vi "Main_v5.vi"() -> ()   [LabVIEW 2018]
uses:
  Clusters/FileDataChannel.ctl
  <vilib>/Platform/TimedLoop/XDataNode/timing_clust.ctl
  <vilib>/Platform/TimedLoop/XDataNode/nitl_modes.ctl
  <vilib>/Platform/TimedLoop/XDataNode/wakeup.ctl
  <vilib>/Analysis/Matrix/Datatypes/RealMatrix.ctl
  Clusters/ArrayPairs.ctl
  Clusters/SwapArrayCluster.ctl
  Clusters/RoscoParams.ctl
  Clusters/SimulationConstants.ctl
  Clusters/SwapIndexes.ctl
  <vilib>/Utility/file.llb/Read Delimited Spreadsheet (DBL).vi
  <vilib>/platform/TimedLoop/XDataNode/XDataNode.xnode
  <vilib>/Platform/TimedLoop/XDataNode/XDNodeRunTimeDep.lvlib
  <vilib>/Analysis/Matrix/NI_Matrix.lvlib
  <vilib>/ptbypt/NI_PtbyPt.lvlib
panel:
  out "error":i32
  in  "Config File Location":path=path "/home/lvuser/testcopy"
  out "Iteration Duration":i64
  out "Generator Speed (rad/s)":sgl(slide)=7.06858e-05 scale=-4.0..4.0
  in  "?":T1(tab)
  out "Generator Speed":sgl(graph)
  out "Torque Setpoint (Nm)":sgl(graph)
  out "Pitch Setpoint":sgl(graph)
  out "Aero Torque":dbl(graph)
  in  "GenSpeed Mean":sgl=10.0
  in  "GenSpeeed Amplitude":sgl=1.0
  out "windspeed":sgl(graph)
  out "Cp 2":dbl
  in  "GenSpeed Mean 2":sgl=3.0
  in  "GenSpeeed Amplitude 2":sgl=7.0
  out "Aero Torque  2":sgl(graph)
  in  "To VS_ControlMode":T2(ring)
  in  "Edit DISCON":bool
  out "DISCON.IN Contents":string
  in  "From VS_ControlMode":T2(ring)
  out "avrSWAP":sgl[](array[numeric])
  out "?":dbl
  out "Disp":dbl
  out "OUT_AEROTQ":sgl
  out "Cp array":dbl[][](array[numeric])
  out "Cp":dbl
  out "OUT_ROTSP":sgl
  out "OUT_DEBUG":sgl
  out "y(t)":dbl[](array[numeric]) format="%#_13g"
  out "thetadotdot/acc":dbl
  out "thetadot/vel":dbl
  out "Rotor Speed (rad/s)":sgl(slide)=7.06858e-05 scale=-4.0..4.0
  out "Torque Setpoint (kNm)":sgl(knob) scale=0.0..21586451.0
  out "Pitch Setpoint":sgl(knob) scale=0.0..1.5
  out "Power (kW)":sgl(slide) scale=0.0..20000000.0 scale format="%.2f"
  in  "Init WindSpeed(m/s)":sgl=7.0
  in  "File path":path=path "/home/lvuser/rosco-tests"
  out "SimLoop Late?":bool
  out "FIFO Loop Late?":bool
  in  "Base filename":string="rosco-tests"
  out "Writing to cRIO?":bool
  in  "WriteData":bool
  in  "?":T3
  out "#RT FIFO":u32
  out "Call to Rosco Failed?":bool
  out "Rosco Return Message":string
  in  "?":bool
  out "time(s)":dbl
  out "RT Loop Late?":bool
  # "FOCAL Realtime Control (IEA 15MW)"
  # "SENSOR INPUTS"
  # "FILEWRITING SETTINGS"
  # "ERRORS"
  # "TURBINE SPECIFICATIONS"
  # "ROSCO OUTPUTS"
  # "RATED POWER: 15000000 W"
  # "RATED TORQUE: 19624046.66 Nm"
  # "RATED GEN SPEED: 0.79168 rad/s"
  # "ROSCO INPUTS"
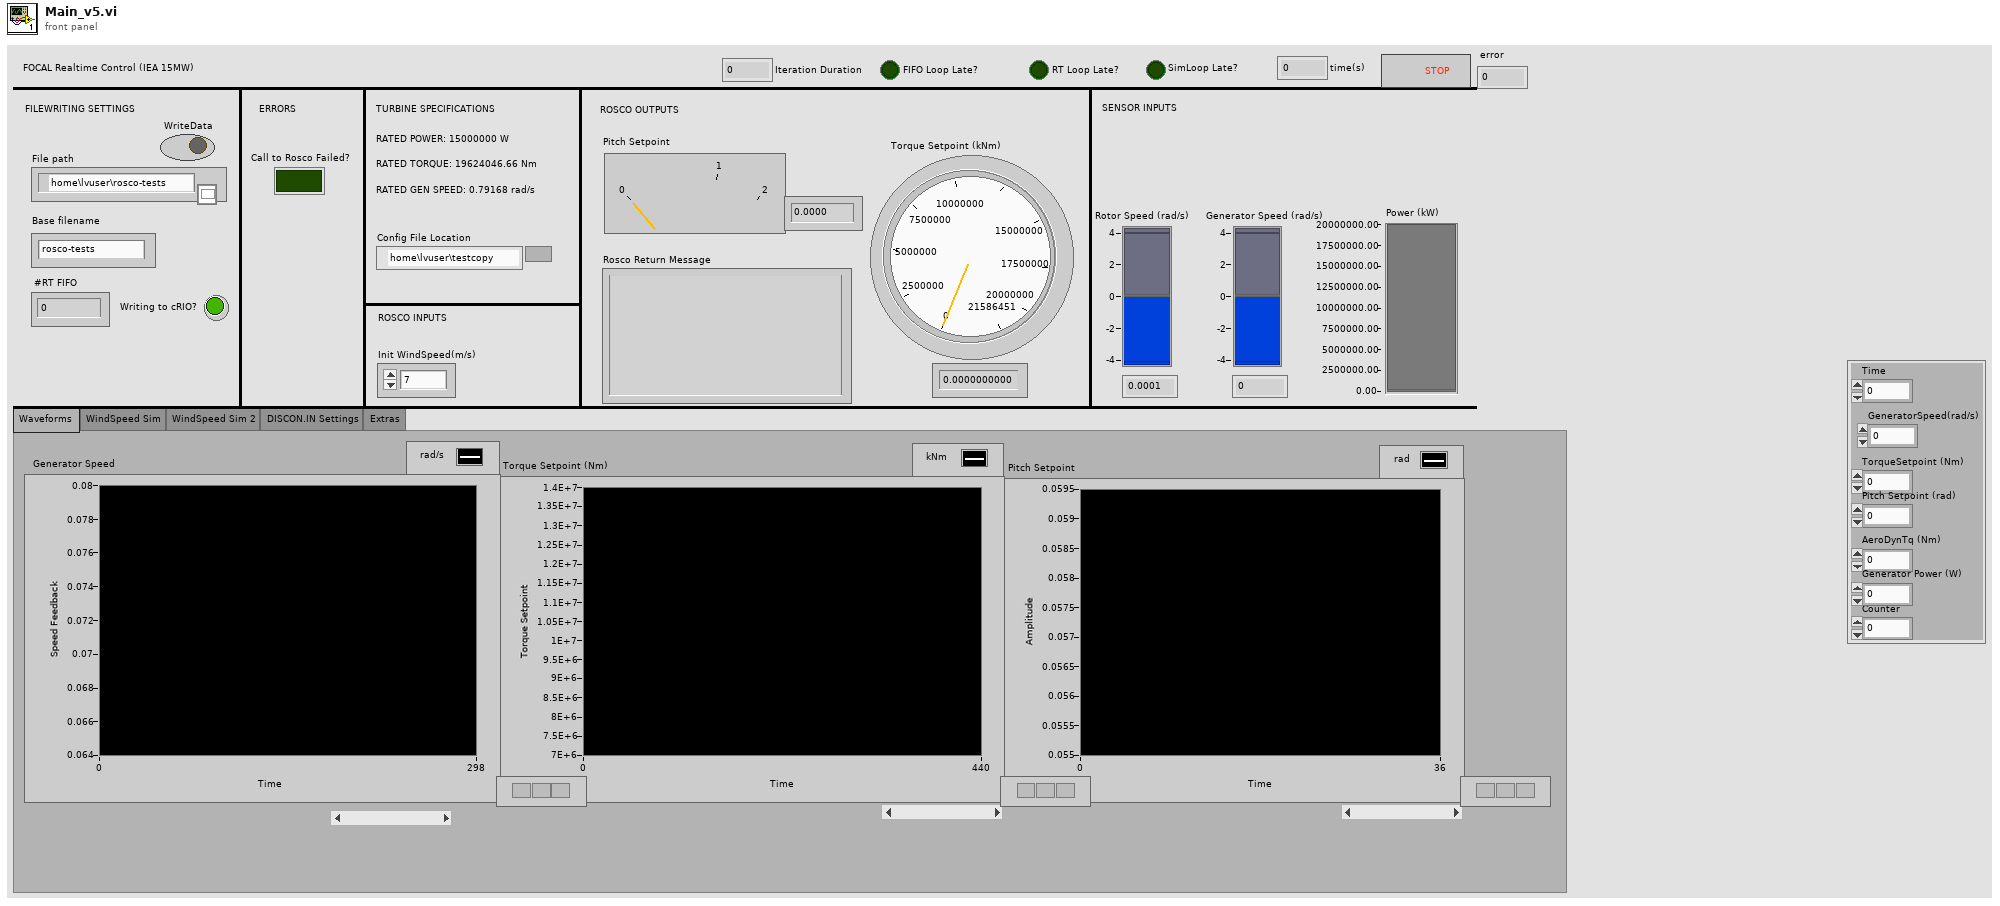
[diagram p1: front panel]
types:
  T1 = enum32{"Waveforms", "WindSpeed Sim", "WindSpeed Sim 2", "DISCON.IN Settings", "Extras"}
  T2 = enum16{"Constant Torque", "Constant Power", "PI Control"}
  T3 = typedef "FileDataChannel.ctl" = cluster{"GeneratorSpeed(rad/s)":sgl, "Counter":sgl, "Time":sgl, "TorqueSetpoint (Nm)":sgl, "Pitch Setpoint (rad)":sgl, "AeroDynTq (Nm) ":sgl, "Generator Power (W) ":sgl}
  T4 = typedef "NI_Matrix.lvlib/RealMatrix.ctl" = dbl[][]
  T5 = typedef "ArrayPairs.ctl" = cluster{"iStatus":T6, "TIME":T6, "DT":T6, "BL_PITCH":T6, "VS_MECHGENPWR":T6, "VS_GENPWR":T6, "GEN_SPEED":T6, "ROTOR_SPEED":T6, "GENTQMEAS":T6, "Y_M":T6, "HORWINDV":T6, "ROOTMOOP1":T6, "ROOTMOOP2":T6, "BL_PITCH2":T6, "BL_PITCH3":T6, "ROOTMOOP3":T6, "AVCMSG_SIZE":T6, "INFILE_SIZE ":T6, "OUTFILE_SIZE ":T6, "FA_ACC":T6, "NUM_BLADES":T6, "OUT_BL_PITCH":T6, "OUT_TORQUE":T6, "OUT_AEROTQ":T6, "Out.RotSpeed ":T6, "Out.DEBUG":T6}
  T6 = typedef "SwapArrayCluster.ctl" = cluster{"Index":i32, "Value":sgl}
  T7 = typedef "RoscoParams.ctl" = cluster{"avrSWAP":sgl[], "aviFAIL":i32, "avcMSG":string, "ReturnValue":i32}
  T8 = typedef "SwapIndexes.ctl" = cluster{"iSTATUS":i32, "TIME":i32, "DT":i32, "BL_PITCH_1":i32, "VS_MECHGENPWR":i32, "GEN_SPEED":i32, "ROT_SPEED":i32, "GENTQMEAS":i32, "Y_M":i32, "HORWINDV":i32, "ROOTMOOP1":i32, "ROOTMOOP2":i32, "BL_PITCH_2":i32, "BL_PITCH_3":i32, "ROOTMOOP3":i32, "INFILE_SIZE":i32, "FA_ACC":i32, "NUM_BLADES":i32, " OUT BL_PITCH":i32, "OUT_ TORQUE":i32, "OUTFILE_SIZE ":i32, "AVCMSG_SIZE":i32, "AERODYN TQ":i32, "VS_GENPWR":i32}
  T9 = typedef "XDNodeRunTimeDep.lvlib/timing_clust.ctl" = cluster{"Expected End [f-1]":u64, "Actual End [f-1]":u64, "Finished Late? [f-1]":bool, "Expected End [i-1]":u64, "Actual End [i-1]":u64, "Finished Late? [i-1]":bool, "Expected Start [i]":u64, "Actual Start [i]":u64, "Expected Start [f]":u64, "Actual Start [f]":u64, "Source Name":string, "Structure Name":string, "Period":i64, "Deadline":i64, "Offset":i64, "Start":i64, "Priority":i32, "Timeout":i32, "Mode":T10, "Wakeup Reason":T11, "Error":errorcluster, "Source Type":string, "Secondary Source Type":string, "Global End Time":u64, "Global Start Time":u64, "Frame Duration":u64, "Iteration Duration":u64, "Assigned CPU":i32, "I/O Scan Engine Mode":u32}
  T10 = typedef "XDNodeRunTimeDep.lvlib/nitl_modes.ctl" = enum32{"No Change", "Process missed periods, maintain original phase", "Discard missed periods, maintain original phase", "Process missed periods, ignore original phase", "Discard missed periods, ignore original phase"}
  T11 = typedef "XDNodeRunTimeDep.lvlib/wakeup.ctl" = enum32{"Normal", "Aborted", "Asynchronous wakeup", "Timing source error", "Timed loop error", "Timeout"}
  T12 = typedef "SimulationConstants.ctl" = cluster{"Ngear":sgl, "RotorInertia":sgl, "GeneratorEff":sgl, "RotorRadius":sgl, "Rho":sgl}
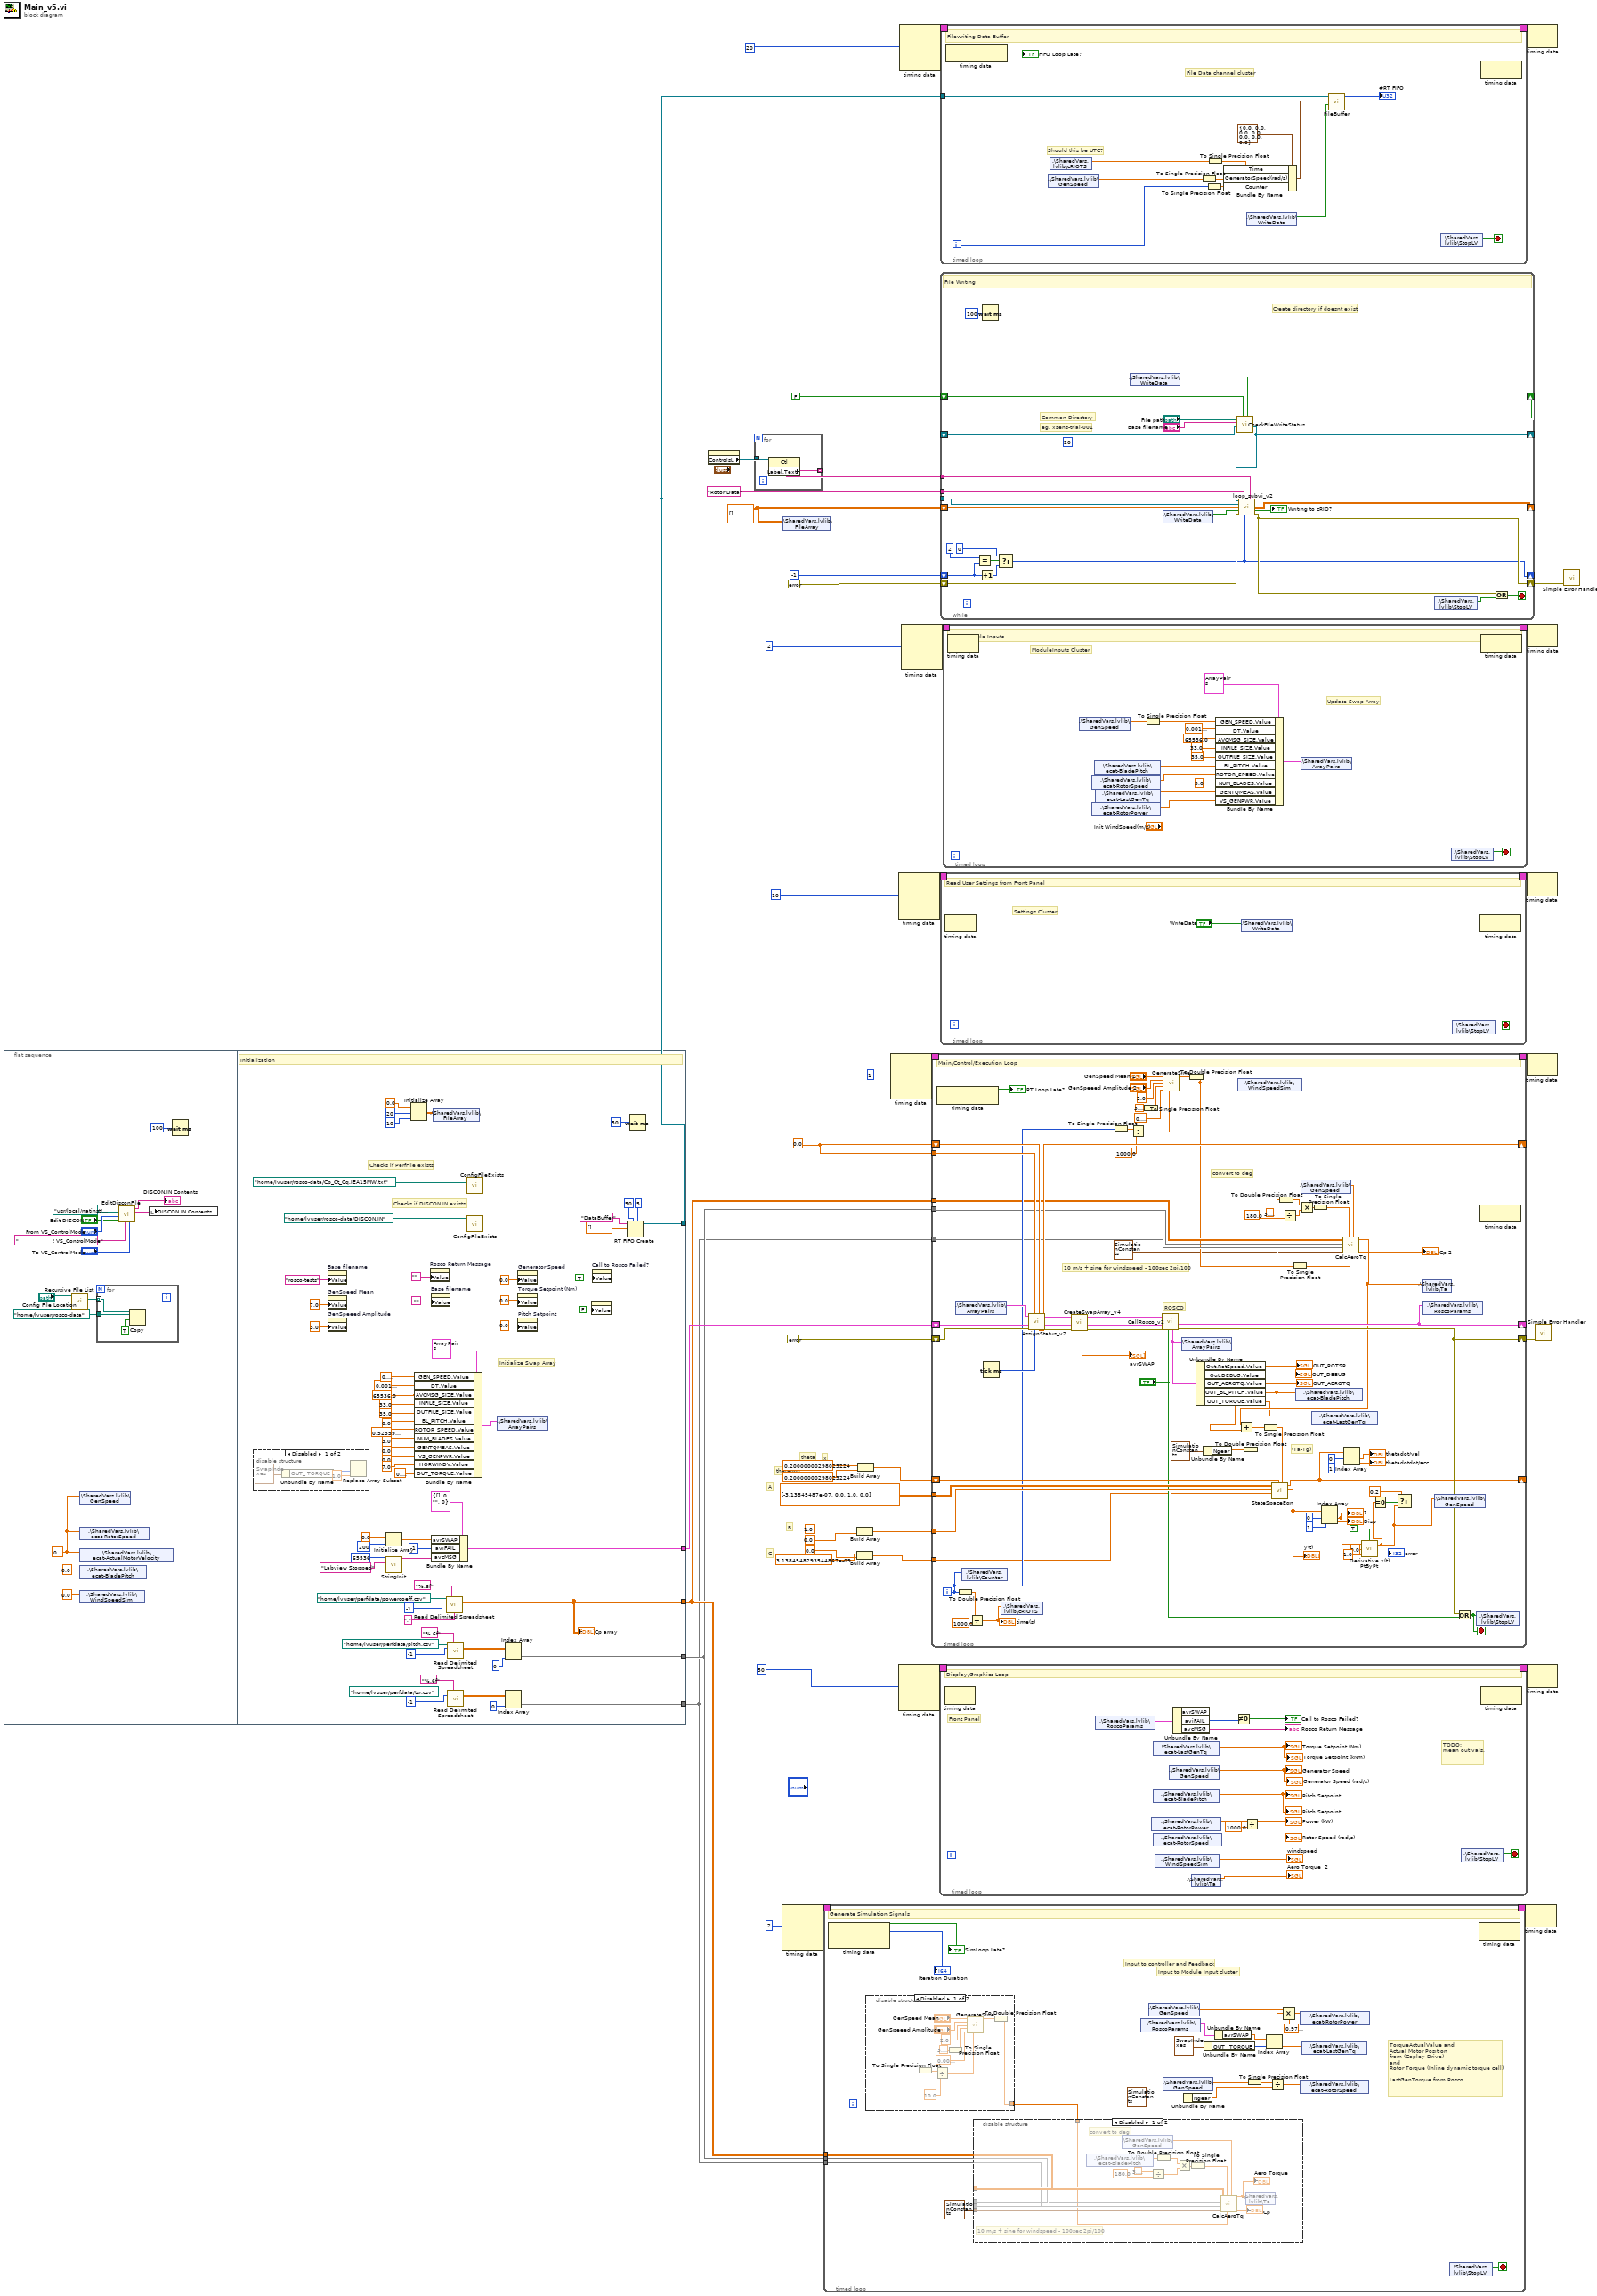
[diagram p0: block diagram]
diagram:
  w21 = dbl[][] [] ("File array 2")
  w28 = 0.0 ("y")
  (unwired) i64 20 ("Period")
  # "thetadot"
  # "theta"
  # "A"
  # "B"
  # "C"
  # "x"
  n1 = flat-sequence {
    tunnel: [w114] -> w22
    tunnel: [w99] -> w14
    tunnel: [w74] -> w8
    tunnel: [w88] -> w7
    tunnel: [w87] -> w6
    frame #0 {
      w49 = sgl 0.2 ("RotorSpeed(rad/s)")
      n2 = call <vilib>:"Recursive File List.vi"("Folder Path"="Config File Location") -> ("All Files in Dir"=w46:path[])  [unwired: 6 in, 4 out]
      n3 = shared-variable ".\\SharedVars.lvlib\\GenSpeed"(w49) -> ()  [unwired: 1 in, 1 out]
      n4 = shared-variable ".\\SharedVars.lvlib\\ecat-RotorSpeed"(w49) -> ()  [unwired: 1 in, 1 out]
      n5 = shared-variable ".\\SharedVars.lvlib\\ecat-ActualMotorVelocity"(w49) -> ()  [unwired: 1 in, 1 out]
      n6 = shared-variable ".\\SharedVars.lvlib\\ecat-BladePitch"(sgl 0.0 ("ecat-BladePitch")) -> ()  [unwired: 1 in, 1 out]
      n7 = shared-variable ".\\SharedVars.lvlib\\WindSpeedSim"(0.0 ("WindSpeedSim")) -> ()  [unwired: 1 in, 1 out]
      n8 = for {
        tunnel: path "/home/lvuser/rosco-data" ("target path (use dialog)") -> [w61]
        tunnel: w46 -> [w60] mode=indexing
        n9 = Copy(9:TRUE ("overwrite (F)"), 10:w61, 11:w60) -> ()  [unwired: 2 in, 3 out]
      }
      n10 = call "EditDisconFile.vi"("To VS_ControlMode"="To VS_ControlMode", "Append"="                   ! VS_ControlMode", "Edit DISCON"="Edit DISCON", "From VS_ControlMode"="From VS_ControlMode", "path"=path "/usr/local/natinst/labview/DISCON.IN") -> ("result string"=w52:string, "data"=→"DISCON.IN Contents":string)  [unwired: 4 in]
      n11 = local write "DISCON.IN Contents"(w52) -> ()
      n12 = Wait (ms)(milliseconds to wait=u32 100) -> ()  [unwired: 1 out]
    }
    frame #1 {
      # "Checks if PerfFile exists"
      # "Checks if DISCON.IN exists"
      # "Initialize Swap Array"
      # "Initialization"
      n13 = disable-structure shown="Disabled" {
        frame Disabled {
          n14 = Unbundle By Name(T8 {"iSTATUS"=0, "TIME"=1, "DT"=2, "BL_PITCH_1"=3, "VS_MECHGENPWR"=13, "GEN_SPEED"=19, "ROT_SPEED"=20, "GENTQMEAS"=22, "Y_M"=23, "HORWINDV"=26, "ROOTMOOP1"=29, "ROOTMOOP2"=30, "BL_PITCH_2"=32, "BL_PITCH_3"=33, "ROOTMOOP3"=31, "INFILE_SIZE"=49, "FA_ACC"=52, "NUM_BLADES"=60, " OUT BL_PITCH"=44, "OUT_ TORQUE"=46, "OUTFILE_SIZE "=50, "AVCMSG_SIZE"=48, "AERODYN TQ"=89, "VS_GENPWR"=14} ("Index In")) -> ("OUT_ TORQUE"=w125:i32)
          n15 = Replace Array Subset(new element=1.0 ("new element/subarray"), index=w125) -> ()  [unwired: 1 in, 1 out]
        }
        frame Enabled {
        }
      }
      n16 = property on="Base filename" class="Str"("Value"="rosco-tests" ("Base filename")) -> ()  [unwired: 2 in, 2 out]
      n17 = property on="GenSpeed Mean" class="DigNum (strict)"("Value"=sgl 7.0 ("GenSpeed Mean")) -> ()  [unwired: 2 in, 2 out]
      n18 = property on="GenSpeeed Amplitude" class="DigNum (strict)"("Value"=sgl 3.0 ("GenSpeeed Amplitude")) -> ()  [unwired: 2 in, 2 out]
      n19 = Initialize Array(sgl 0.0 ("element"), 200 ("dimension size")) -> (w67:sgl[])
      n20 = call "StringInit.vi"("accOUTNAME"="Labview Stopped", "dimension size"=65536) -> ("result string"=w118:string)  [unwired: 9 in]
      n21 = Initialize Array(0.0 ("element"), 20 ("dimension size"), 10 ("dimension size")) -> (w110:dbl[][])
      n22 = Bundle By Name(cluster=T5 {"iStatus"={"Index"=0, "Value"=0.0}, "TIME"={"Index"=1, "Value"=0.0}, "DT"={"Index"=2, "Value"=0.0}, "BL_PITCH"={"Index"=3, "Value"=0.0}, "VS_MECHGENPWR"={"Index"=13, "Value"=0.0}, "VS_GENPWR"={"Index"=14, "Value"=0.0}, "GEN_SPEED"={"Index"=19, "Value"=0.0}, "ROTOR_SPEED"={"Index"=20, "Value"=0.0}, "GENTQMEAS"={"Index"=22, "Value"=0.0}, "Y_M"={"Index"=23, "Value"=0.0}, "HORWINDV"={"Index"=26, "Value"=0.0}, "ROOTMOOP1"={"Index"=29, "Value"=0.0}, "ROOTMOOP2"={"Index"=30, "Value"=0.0}, "BL_PITCH2"={"Index"=32, "Value"=0.0}, "BL_PITCH3"={"Index"=33, "Value"=0.0}, "ROOTMOOP3"={"Index"=31, "Value"=0.0}, "AVCMSG_SIZE"={"Index"=48, "Value"=0.0}, "INFILE_SIZE "={"Index"=49, "Value"=0.0}, "OUTFILE_SIZE "={"Index"=50, "Value"=0.0}, "FA_ACC"={"Index"=52, "Value"=0.0}, "NUM_BLADES"={"Index"=60, "Value"=0.0}, "OUT_BL_PITCH"={"Index"=44, "Value"=0.0}, "OUT_TORQUE"={"Index"=46, "Value"=0.0}, "OUT_AEROTQ"={"Index"=91, "Value"=0.0}, "Out.RotSpeed "={"Index"=92, "Value"=0.0}, "Out.DEBUG"={"Index"=93, "Value"=0.0}} ("ArrayPairs"), "GEN_SPEED.Value"=sgl 0.3 ("GeneratorSpeed(rad/s)"), "DT.Value"=sgl 0.001 ("Dt"), "AVCMSG_SIZE.Value"=sgl 65536.0 ("new element/subarray"), "INFILE_SIZE.Value"=sgl 33.0 ("new element/subarray"), "OUTFILE_SIZE.Value"=sgl 35.0 ("new element/subarray"), "BL_PITCH.Value"=sgl 0.0 ("GeneratorTorque(Nm)"), "ROTOR_SPEED.Value"=sgl 0.5236 ("RotorSpeed(rad/s)"), "NUM_BLADES.Value"=sgl 3.0 ("NumberofBlades"), "GENTQMEAS.Value"=sgl 0.0 ("BladePitch(rad)"), "VS_GENPWR.Value"=sgl 0.0 ("Generator Power(W)"), "HORWINDV.Value"=sgl 7.0 ("WindSpeed(m/s)"), "OUT_TORQUE.Value"=sgl 0.2) -> (w75:T5)
      n23 = property on="Rosco Return Message" class="Str"("Value"="") -> ()  [unwired: 2 in, 2 out]
      n24 = property on="Base filename" class="Str"("Value"="") -> ()  [unwired: 2 in, 2 out]
      n25 = Bundle By Name(cluster=T7 {"avrSWAP"=[], "aviFAIL"=0, "avcMSG"="", "ReturnValue"=0}, "avrSWAP"=w67, "aviFAIL"=-1, "avcMSG"=w118) -> (w99:T7)
      n26 = shared-variable ".\\SharedVars.lvlib\\FileArray"(w110) -> ()  [unwired: 1 in, 1 out]
      n27 = call-poly <vilib>:"Read Delimited Spreadsheet.vi"("file path (dialog if empty)"=path "/home/lvuser/perfdata/powercoeff.csv", "format (%.3f)"="%.6f", "number of rows (all:-1)"=-1, "delimiter (\\t)"="," ("delimiter (\\t)")) -> ("all rows"=w74:dbl[][])  [unwired: 6 in, 5 out]
      "Cp array" <- w74
      n28 = call-poly <vilib>:"Read Delimited Spreadsheet.vi"("file path (dialog if empty)"=path "/home/lvuser/perfdata/pitch.csv", "format (%.3f)"="%.6f", "number of rows (all:-1)"=-1) -> ("all rows"=w92:dbl[][])  [unwired: 7 in, 5 out]
      n29 = call-poly <vilib>:"Read Delimited Spreadsheet.vi"("file path (dialog if empty)"=path "/home/lvuser/perfdata/tsr.csv", "format (%.3f)"="%.6f", "number of rows (all:-1)"=-1) -> ("all rows"=w94:dbl[][])  [unwired: 7 in, 5 out]
      n30 = call "ConfigFileExists.vi"("path"=path "/home/lvuser/rosco-data/Cp_Ct_Cq.IEA15MW.txt") -> ()  [unwired: 11 in]
      n31 = call "ConfigFileExists.vi"("path"=path "/home/lvuser/rosco-data/DISCON.IN") -> ()  [unwired: 11 in]
      n32 = shared-variable ".\\SharedVars.lvlib\\ArrayPairs"(w75) -> ()  [unwired: 1 in, 1 out]
      n33 = Index Array(array=w92, index (col)=0 ("disabled index (col)")) -> (element=w88:dbl[])  [unwired: 1 in]
      n34 = Index Array(array=w94, index (col)=0 ("disabled index (col)")) -> (element=w87:dbl[])  [unwired: 1 in]
      n35 = property on="Generator Speed" class="WFChart (strict)"("Value"=sgl 0.0 ("Generator Speed")) -> ()  [unwired: 2 in, 2 out]
      n36 = property on="Torque Setpoint (Nm)" class="WFChart (strict)"("Value"=sgl 0.0 ("Generator Speed")) -> ()  [unwired: 2 in, 2 out]
      n37 = property on="Pitch Setpoint" class="WFChart (strict)"("Value"=sgl 0.0 ("Generator Speed")) -> ()  [unwired: 2 in, 2 out]
      n38 = property class="Bool (strict)"("Value"=FALSE) -> ()  [unwired: 2 in, 2 out]
      n39 = property on="Call to Rosco Failed?" class="Bool (strict)"("Value"=TRUE ("Call to Rosco Failed?")) -> ()  [unwired: 2 in, 2 out]
      n40 = RT FIFO Create(0:"DataBuffer" ("name (unnamed)"), 1:dbl[] [] ("appended array"), 4:u32 50, 6:u32 5) -> (8:w114:refnum<k33>)  [unwired: 4 in, 2 out]
      n41 = Wait (ms)(milliseconds to wait=u32 50) -> ()  [unwired: 1 out]
    }
  }
  n42 = property class="Clust (strict)"() -> ("Controls[]"=w25:refnum<vi>[])  [unwired: 2 in, 2 out]
  n43 = for {
    tunnel: w25 -> [w128] mode=indexing
    tunnel: [w127] -> w24 mode=indexing
    n44 = property class="Ctl"(reference=w128) -> ("Label.Text"=w127:string)  [unwired: 1 in, 2 out]
  }
  n45 = node-c288(i64 2 ("Period")) -> (w36:T9)  [unwired: 3 in]
  n46 = shared-variable ".\\SharedVars.lvlib\\FileArray"(w21) -> ()  [unwired: 1 in, 1 out]
  n47 = timed-loop {
    timing: w36 -> [_]
    timing-out: [_] -> w35
    tunnel: w8 -> [w146]
    tunnel: w7 -> [w145]
    tunnel: w6 -> [w144]
    stop <- w149 stop-if-true
    # "TorqueActualValue and \nActual Motor Position \nfrom (Copley Drive)\nand\nRotor Torque (Inline dynamic torque cell)\n\nLastGenTorque from Rosco"
    # "Input to Module Input cluster"
    # "Input to controller and Feedback"
    # "Generate Simulation Signals"
    n48 = node-c288() -> (→"SimLoop Late?":bool, →"Iteration Duration":i64)  [unwired: 1 in]
    n49 = disable-structure shown="Disabled" {
      disable-tunnel: [w165 _] -> w142
      frame Disabled {
        n50 = To Single Precision Float() -> (single precision float=w175:sgl)  [unwired: 1 in]
        n51 = Divide(x=w175, y=sgl 10.0) -> (x/y=w169:sgl)
        n52 = To Single Precision Float(number=3.141592653589793 ("value")) -> (single precision float=w167:sgl)
        n53 = call "GenerateSine.vi"("GenSpeed Mean"="GenSpeed Mean", "GenSpeeed Amplitude"="GenSpeeed Amplitude", "2"=sgl 2.0 ("value"), "pi"=w167, "frequency (f)"=sgl 0.01 ("value"), "time (s)"=w169) -> ("sine out"=w166:sgl)  [unwired: 9 in]
        n54 = To Double Precision Float(number=w166) -> (double precision float=w165:dbl)
      }
      frame Enabled {
      }
    }
    n55 = disable-structure shown="Disabled" {
      disable-tunnel: w146 -> [w164 _]
      disable-tunnel: w145 -> [w163 _]
      disable-tunnel: w144 -> [w162 _]
      disable-tunnel: T12 {"Ngear"=1.0, "RotorInertia"=318628130.0, "GeneratorEff"=0.97, "RotorRadius"=0.97, "Rho"=0.97} ("SimulationConst") -> [w161 _]
      disable-tunnel: w142 -> [w158 _]
      frame Disabled {
        # "convert to deg"
        # "10 m/s + sine for windspeed - 100sec 2pi/100"
        n56 = shared-variable ".\\SharedVars.lvlib\\ecat-BladePitch"() -> (w154:sgl)  [unwired: 1 in, 1 out]
        n57 = shared-variable ".\\SharedVars.lvlib\\GenSpeed"() -> (w157:sgl)  [unwired: 1 in, 1 out]
        n58 = Divide(x=3.141592653589793, y=180.0) -> (x/y=w153:dbl)
        n59 = To Double Precision Float(number=w154) -> (double precision float=w152:dbl)
        n60 = Multiply(x=w152, y=w153) -> (x*y=w151:dbl)
        n61 = To Single Precision Float(number=w151) -> (single precision float=w150:sgl)
        n62 = call "CalcAeroTq.vi"("GenSpeed"=w157, "WindSpeed"=w158, "Xi"=w150, "SimulationConst"=w161, "tsr(Y)"=w162, "pitch (X)"=w163, "Cp(Z)"=w164) -> ("Cp"=→"Cp":dbl, "Ta"=w159:dbl)  [unwired: 2 in]
        "Aero Torque" <- w159
        n63 = shared-variable ".\\SharedVars.lvlib\\Ta"(w159) -> ()  [unwired: 1 in, 1 out]
      }
      frame Enabled {
      }
    }
    n64 = shared-variable ".\\SharedVars.lvlib\\RoscoParams"() -> (w135:T7)  [unwired: 1 in, 1 out]
    n65 = shared-variable ".\\SharedVars.lvlib\\GenSpeed"() -> (w136:sgl)  [unwired: 1 in, 1 out]
    n66 = shared-variable ".\\SharedVars.lvlib\\GenSpeed"() -> (w132:sgl)  [unwired: 1 in, 1 out]
    n67 = Unbundle By Name(T12 {"Ngear"=1.0, "RotorInertia"=318628130.0, "GeneratorEff"=0.97, "RotorRadius"=120.0, "Rho"=1.225} ("SimulationConst")) -> ("Ngear"=w134:sgl)
    n68 = Unbundle By Name(T8 {"iSTATUS"=0, "TIME"=1, "DT"=2, "BL_PITCH_1"=3, "VS_MECHGENPWR"=13, "GEN_SPEED"=19, "ROT_SPEED"=20, "GENTQMEAS"=22, "Y_M"=23, "HORWINDV"=26, "ROOTMOOP1"=29, "ROOTMOOP2"=30, "BL_PITCH_2"=32, "BL_PITCH_3"=33, "ROOTMOOP3"=31, "INFILE_SIZE"=49, "FA_ACC"=52, "NUM_BLADES"=60, " OUT BL_PITCH"=44, "OUT_ TORQUE"=46, "OUTFILE_SIZE "=50, "AVCMSG_SIZE"=48, "AERODYN TQ"=89, "VS_GENPWR"=14} ("Index In")) -> ("OUT_ TORQUE"=w137:i32)
    n69 = Unbundle By Name(w135) -> ("avrSWAP"=w138:sgl[])
    n70 = To Single Precision Float(number=w132) -> (single precision float=w131:sgl)
    n71 = Index Array(array=w138, index=w137) -> (element=w141:sgl)
    n72 = Divide(x=w131, y=w134) -> (x/y=w133:sgl)
    n73 = Compound Arithmetic op=MULTIPLY(w136, w141, sgl 0.97 ("value")) -> (w139:sgl)
    n74 = shared-variable ".\\SharedVars.lvlib\\ecat-RotorPower"(w139) -> ()  [unwired: 1 in, 1 out]
    n75 = shared-variable ".\\SharedVars.lvlib\\ecat-RotorSpeed"(w133) -> ()  [unwired: 1 in, 1 out]
    n76 = shared-variable ".\\SharedVars.lvlib\\ecat-LastGenTq"(w141) -> ()  [unwired: 1 in, 1 out]
    n77 = shared-variable ".\\SharedVars.lvlib\\StopLV"() -> (w149:bool)  [unwired: 1 in, 1 out]
    n78 = node-c288() -> ()  [unwired: 1 in, 1 out]
  }
  n79 = Build Array(sgl 1.0 ("element"), sgl 0.0 ("element")) -> (w5:sgl[])
  n80 = Build Array(sgl 3.1384548e-09 ("element"), sgl 0.0 ("element")) -> (w4:sgl[])
  n81 = Build Array(sgl 0.2 ("element"), sgl 0.2 ("element")) -> (w11:sgl[])
  n82 = node-c288(i64 1 ("Period")) -> (w34:T9)  [unwired: 3 in]
  n83 = node-c288(i64 50 ("Period")) -> (w38:T9)  [unwired: 3 in]
  n84 = node-c288(i64 10 ("Period")) -> (w40:T9)  [unwired: 3 in]
  n85 = node-c288(i64 20 ("Period")) -> (w44:T9)  [unwired: 3 in]
  n86 = node-c288(i64 2 ("Period")) -> (w42:T9)  [unwired: 3 in]
  n87 = timed-loop {
    timing: w34 -> [_]
    timing-out: [_] -> w33
    shift-right: [w242] -> _
    shift-left: w28 -> [w244]
    tunnel: w28 -> [w243]
    shift-right: [w233] -> _
    shift-left: w14 -> [w247]
    shift-right: [w234] -> w15
    shift-left: errorcluster {"status"=FALSE, "code"=0, "source"=""} ("error out") -> [w246]
    shift-right: [w193] -> _
    shift-left: w11 -> [w253]
    tunnel: T4 [[-3.13845487e-07, 0.0], [1.0, 0.0]] ("A") -> [w252]
    tunnel: w5 -> [w251]
    tunnel: w8 -> [w206]
    tunnel: w7 -> [w205]
    tunnel: w6 -> [w204]
    tunnel: w4 -> [w201]
    i -> [w207]
    stop <- w254 stop-if-true
    (unwired) 1 ("index")
    # "(Ta-Tg)"
    # "convert to deg"
    # "10 m/s + sine for windspeed - 100sec 2pi/100"
    # "ROSCO"
    # "Main/Control/Execution Loop"
    n88 = node-c288() -> (→"RT Loop Late?":bool)  [unwired: 1 in]
    n89 = shared-variable ".\\SharedVars.lvlib\\ArrayPairs"() -> (w248:T5)  [unwired: 1 in, 1 out]
    n90 = To Double Precision Float(number=w207) -> (double precision float=w256:dbl)
    n91 = shared-variable ".\\SharedVars.lvlib\\Counter"(w207) -> ()  [unwired: 1 in, 1 out]
    n92 = Divide(x=w256, y=1000.0) -> (x/y=w229:dbl)
    "time(s)" <- w229
    n93 = Tick Count (ms)() -> (millisecond timer value=w245:u32)
    n94 = shared-variable ".\\SharedVars.lvlib\\cRIOTS"(w229) -> ()  [unwired: 1 in, 1 out]
    n95 = call "AssignStatus_v2.vi"("LoopCount"=w244, "Time"=w245, "Init Val"=w243, "error in (no error)"=w246, "ROSCO Params"=w247, "ArrayPairs In"=w248) -> ("error out"=w239:errorcluster, "ROSCO Params 2"=w240:T7, "ArrayPairs Out"=w241:T5, "Count+1"=w242:dbl)  [unwired: 2 in]
    n96 = call "CreateSwapArray_v4.vi"("error in (no error)"=w239, "ROSCO Params"=w240, "ArrayPairs"=w241) -> ("error out"=w235:errorcluster, "ROSCO Params Out"=w236:T7, "ArrayPairs Out"=w237:T5, "avrSWAP"=→"avrSWAP":sgl[])  [unwired: 5 in]
    n97 = To Single Precision Float(number=w207) -> (single precision float=w223:sgl)
    n98 = Divide(x=w223, y=sgl 1000.0) -> (x/y=w217:sgl)
    n99 = To Single Precision Float(number=3.141592653589793 ("value")) -> (single precision float=w215:sgl)
    n100 = call "CallRosco_v2.vi"("StopLV"="?", "error in (no error)"=w235, "ROSCO Params in"=w236, "ArrayPairs"=w237) -> ("error out"=w234:errorcluster, "ROSCO Params out"=w233:T7, "ArrayPairs 2"=w231:T5)  [unwired: 5 in]
    n101 = call "GenerateSine.vi"("GenSpeed Mean"="GenSpeed Mean 2", "GenSpeeed Amplitude"="GenSpeeed Amplitude 2", "2"=sgl 2.0 ("value"), "pi"=w215, "frequency (f)"=sgl 0.1 ("value"), "time (s)"=w217) -> ("sine out"=w214:sgl)  [unwired: 9 in]
    n102 = shared-variable ".\\SharedVars.lvlib\\ArrayPairs"(w231) -> ()  [unwired: 1 in, 1 out]
    n103 = To Double Precision Float(number=w214) -> (double precision float=w200:dbl)
    n104 = Unbundle By Name(w231) -> ("Out.RotSpeed.Value"=→"OUT_ROTSP":sgl, "Out.DEBUG.Value"=→"OUT_DEBUG":sgl, "OUT_AEROTQ.Value"=→"OUT_AEROTQ":sgl, "OUT_BL_PITCH.Value"=w199:sgl, "OUT_TORQUE.Value"=w191:sgl)
    n105 = Unbundle By Name(T12 {"Ngear"=1.0, "RotorInertia"=318628130.0, "GeneratorEff"=0.97, "RotorRadius"=120.0, "Rho"=1.225} ("SimulationConst")) -> ("Ngear"=w228:sgl)
    n106 = shared-variable ".\\SharedVars.lvlib\\WindSpeedSim"(w200) -> ()  [unwired: 1 in, 1 out]
    n107 = To Double Precision Float(number=w228) -> ()  [unwired: 1 out]
    n108 = To Double Precision Float(number=w199) -> (double precision float=w210:dbl)
    n109 = Divide(x=3.141592653589793, y=180.0) -> (x/y=w211:dbl)
    n110 = To Single Precision Float(number=w200) -> (single precision float=w198:sgl)
    n111 = shared-variable ".\\SharedVars.lvlib\\ecat-BladePitch"(w199) -> ()  [unwired: 1 in, 1 out]
    n112 = Multiply(x=w210, y=w211) -> (x*y=w209:dbl)
    n113 = shared-variable ".\\SharedVars.lvlib\\GenSpeed"() -> (w195:sgl)  [unwired: 1 in, 1 out]
    n114 = shared-variable ".\\SharedVars.lvlib\\ecat-LastGenTq"(w191) -> ()  [unwired: 1 in, 1 out]
    n115 = To Single Precision Float(number=w209) -> (single precision float=w208:sgl)
    n116 = call "CalcAeroTq.vi"("GenSpeed"=w195, "WindSpeed"=w198, "Xi"=w208, "SimulationConst"=T12 {"Ngear"=1.0, "RotorInertia"=318628130.0, "GeneratorEff"=0.97, "RotorRadius"=120.0, "Rho"=1.225}, "tsr(Y)"=w204, "pitch (X)"=w205, "Cp(Z)"=w206) -> ("Cp"=→"Cp 2":dbl, "Ta"=w202:dbl)  [unwired: 2 in]
    n117 = Add(x=w202, y=w191) -> (x+y=w203:dbl)
    n118 = To Single Precision Float(number=w203) -> (single precision float=w190:sgl)
    n119 = call "StateSpaceEqn.vi"("u"=w190, "x"=w253, "C"=w201, "B"=w251, "A"=w252) -> ("y(t)"=w225:sgl[], "x(t+1)"=w193:sgl[])  [unwired: 5 in]
    "y(t)" <- w225
    n120 = Index Array(array=w225, index #1=0 ("index"), index #2=1 ("index")) -> (element #1=w180:sgl, element #2=→"Disp":sgl)
    "?" <- w180
    n121 = Index Array(array=w193, index #1=0 ("index")) -> (element #1=→"thetadot/vel":sgl, element #2=→"thetadotdot/acc":sgl)  [unwired: 1 in]
    n122 = call <vilib>:"Derivative x(t) PtByPt.vi"("initialize"=TRUE, "dt"=1.0, "initial condition"=0.0, "x"=w180) -> ("error"=→"error":i32, "dx/dt"=w183:dbl)
    n123 = Equal To 0?(x=w183) -> (x = 0?=w189:bool)
    n124 = Select(t=0.2, s=w189, f=w183) -> ()  [unwired: 1 out]
    n125 = shared-variable ".\\SharedVars.lvlib\\Ta"(w202) -> ()  [unwired: 1 in, 1 out]
    n126 = shared-variable ".\\SharedVars.lvlib\\RoscoParams"(w233) -> ()  [unwired: 1 in, 1 out]
    n127 = shared-variable ".\\SharedVars.lvlib\\GenSpeed"(w183) -> ()  [unwired: 1 in, 1 out]
    n128 = Or(x=w234, y="?") -> (x .or. y?=w254:bool)
    n129 = shared-variable ".\\SharedVars.lvlib\\StopLV"(w254) -> ()  [unwired: 1 in, 1 out]
    n130 = node-c288() -> ()  [unwired: 1 in, 1 out]
  }
  n131 = timed-loop {
    timing: w38 -> [_]
    timing-out: [_] -> w37
    stop <- w274 stop-if-true
    # "TODO:\nmean out vals."
    # "Front Panel"
    # "Display/Graphics Loop"
    n132 = node-c288() -> ()  [unwired: 1 in, 1 out]
    n133 = shared-variable ".\\SharedVars.lvlib\\RoscoParams"() -> (w273:T7)  [unwired: 1 in, 1 out]
    n134 = shared-variable ".\\SharedVars.lvlib\\ecat-RotorPower"() -> (w269:sgl)  [unwired: 1 in, 1 out]
    n135 = shared-variable ".\\SharedVars.lvlib\\ecat-RotorSpeed"() -> (→"Rotor Speed (rad/s)":sgl)  [unwired: 1 in, 1 out]
    n136 = shared-variable ".\\SharedVars.lvlib\\ecat-LastGenTq"() -> (→"Torque Setpoint (Nm)" →"Torque Setpoint (kNm)":sgl)  [unwired: 1 in, 1 out]
    n137 = shared-variable ".\\SharedVars.lvlib\\ecat-BladePitch"() -> (→"Pitch Setpoint" →"Pitch Setpoint":sgl)  [unwired: 1 in, 1 out]
    n138 = shared-variable ".\\SharedVars.lvlib\\WindSpeedSim"() -> (→"windspeed":sgl)  [unwired: 1 in, 1 out]
    n139 = shared-variable ".\\SharedVars.lvlib\\GenSpeed"() -> (→"Generator Speed" →"Generator Speed (rad/s)":sgl)  [unwired: 1 in, 1 out]
    n140 = Unbundle By Name(w273) -> ("aviFAIL"=w271:i32, "avcMSG"=→"Rosco Return Message":string)  [unwired: 1 out]
    n141 = shared-variable ".\\SharedVars.lvlib\\Ta"() -> (→"Aero Torque  2":sgl)  [unwired: 1 in, 1 out]
    n142 = Not Equal To 0?(x=w271) -> (x != 0?=→"Call to Rosco Failed?":bool)
    n143 = Divide(x=w269, y=sgl 1000.0) -> (x/y=→"Power (kW)":sgl)
    n144 = shared-variable ".\\SharedVars.lvlib\\StopLV"() -> (w274:bool)  [unwired: 1 in, 1 out]
    n145 = node-c288() -> ()  [unwired: 1 in, 1 out]
  }
  n146 = while {
    shift-right: [w277] -> _
    shift-left: _ -> [w278]
    shift-right: [w285] -> _
    shift-left: FALSE -> [w286]
    shift-right: [w298] -> w17
    shift-left: errorcluster {"status"=FALSE, "code"=0, "source"=""} ("error out") -> [w297]
    tunnel: "Rotor Data" -> [w280]
    tunnel: w24 -> [w281]
    tunnel: w22 -> [w282]
    shift-right: [w294] -> _
    shift-left: -1 -> [w296]
    shift-right: [w289] -> _
    shift-left: w21 -> [w295]
    stop <- w300 stop-if-true
    # "eg. xsens-trial-001"
    # "Create directory if doesnt exist"
    # "Common Directory"
    # "File Writing"
    n147 = Equal?(x=2 ("t"), y=w296) -> (x = y?=w291:bool)
    n148 = Increment(x=w296) -> (x+1=w290:i32)
    n149 = Wait (ms)(milliseconds to wait=u32 100) -> ()  [unwired: 1 out]
    n150 = Select(t=0, s=w291, f=w290) -> (s? t:f=w294:i32)
    n151 = shared-variable ".\\SharedVars.lvlib\\WriteData"() -> (w287:bool)  [unwired: 1 in, 1 out]
    n152 = shared-variable ".\\SharedVars.lvlib\\WriteData"() -> (w283:bool)  [unwired: 1 in, 1 out]
    n153 = call "CheckFIleWriteStatus.vi"("WriteDataButtonVal"=w287, "WritePrevVal"=w286, "Refnum in"=w278, "Base filename"="Base filename", "File path"="File path") -> ("Refnum out"=w277:refnum<k34>, "WriteCurrentVal"=w285:bool)  [unwired: 5 in]
    n154 = call "loop_subvi_v2.vi"("Refnum in"=w277, "Group Name"=w280, "Channel Names"=w281, "rt fifo"=w282, "File array"=w295, "Write?"=w283, "error in (no error)"=w297, "index"=w294) -> ("File array 2"=w289:dbl[][], "Writing to file"=→"Writing to cRIO?":bool, "error out"=w298:errorcluster)  [unwired: 4 in, 1 out]
    n155 = shared-variable ".\\SharedVars.lvlib\\StopLV"() -> (w301:bool)  [unwired: 1 in, 1 out]
    n156 = Or(x=w298, y=w301) -> (x .or. y?=w300:bool)
  }
  n157 = timed-loop {
    timing: w40 -> [_]
    timing-out: [_] -> w39
    stop <- w303 stop-if-true
    # "Settings Cluster"
    # "Read User Settings from Front Panel"
    n158 = node-c288() -> ()  [unwired: 1 in, 1 out]
    n159 = shared-variable ".\\SharedVars.lvlib\\WriteData"("WriteData") -> ()  [unwired: 1 in, 1 out]
    n160 = shared-variable ".\\SharedVars.lvlib\\StopLV"() -> (w303:bool)  [unwired: 1 in, 1 out]
    n161 = node-c288() -> ()  [unwired: 1 in, 1 out]
  }
  n162 = timed-loop {
    timing: w44 -> [_]
    timing-out: [_] -> w43
    tunnel: w22 -> [w312]
    i -> [w309]
    stop <- w318 stop-if-true
    # "Should this be UTC?"
    # "File Data channel cluster"
    # "Filewriting Data Buffer"
    n163 = node-c288() -> (→"FIFO Loop Late?":bool)  [unwired: 1 in]
    n164 = shared-variable ".\\SharedVars.lvlib\\GenSpeed"() -> (w317:sgl)  [unwired: 1 in, 1 out]
    n165 = shared-variable ".\\SharedVars.lvlib\\cRIOTS"() -> (w306:dbl)  [unwired: 1 in, 1 out]
    n166 = To Single Precision Float(number=w317) -> (single precision float=w307:sgl)
    n167 = To Single Precision Float(number=w309) -> (single precision float=w310:sgl)
    n168 = To Single Precision Float(number=w306) -> (single precision float=w316:sgl)
    n169 = Bundle By Name(cluster=T3 {"GeneratorSpeed(rad/s)"=0.0, "Counter"=0.0, "Time"=0.0, "TorqueSetpoint (Nm)"=0.0, "Pitch Setpoint (rad)"=0.0, "AeroDynTq (Nm) "=0.0, "Generator Power (W) "=0.0} ("SwapIn"), "Time"=w316, "GeneratorSpeed(rad/s)"=w307, "Counter"=w310) -> (w314:T3)
    n170 = shared-variable ".\\SharedVars.lvlib\\WriteData"() -> (w313:bool)  [unwired: 1 in, 1 out]
    n171 = call "FileBuffer.vi"("Boolean"=w313, "FileDataChannel"=w314, "Refnum in"=w312) -> ("# elements"=→"#RT FIFO":u32)  [unwired: 8 in]
    n172 = shared-variable ".\\SharedVars.lvlib\\StopLV"() -> (w318:bool)  [unwired: 1 in, 1 out]
    n173 = node-c288() -> ()  [unwired: 1 in, 1 out]
  }
  n174 = timed-loop {
    timing: w42 -> [_]
    timing-out: [_] -> w41
    stop <- w335 stop-if-true
    # "Update Swap Array"
    # "ModuleInputs Cluster"
    # "Read Module Inputs"
    n175 = node-c288() -> ()  [unwired: 1 in, 1 out]
    n176 = shared-variable ".\\SharedVars.lvlib\\GenSpeed"() -> (w330:sgl)  [unwired: 1 in, 1 out]
    n177 = shared-variable ".\\SharedVars.lvlib\\ecat-RotorSpeed"() -> (w327:sgl)  [unwired: 1 in, 1 out]
    n178 = shared-variable ".\\SharedVars.lvlib\\ecat-RotorPower"() -> (w324:sgl)  [unwired: 1 in, 1 out]
    n179 = shared-variable ".\\SharedVars.lvlib\\ecat-BladePitch"() -> (w328:sgl)  [unwired: 1 in, 1 out]
    n180 = shared-variable ".\\SharedVars.lvlib\\ecat-LastGenTq"() -> (w325:sgl)  [unwired: 1 in, 1 out]
    n181 = To Single Precision Float(number=w330) -> (single precision float=w329:sgl)
    n182 = Bundle By Name(cluster=T5 {"iStatus"={"Index"=0, "Value"=0.0}, "TIME"={"Index"=1, "Value"=0.0}, "DT"={"Index"=2, "Value"=0.0}, "BL_PITCH"={"Index"=3, "Value"=0.0}, "VS_MECHGENPWR"={"Index"=13, "Value"=0.0}, "VS_GENPWR"={"Index"=14, "Value"=0.0}, "GEN_SPEED"={"Index"=19, "Value"=0.0}, "ROTOR_SPEED"={"Index"=20, "Value"=0.0}, "GENTQMEAS"={"Index"=22, "Value"=0.0}, "Y_M"={"Index"=23, "Value"=0.0}, "HORWINDV"={"Index"=26, "Value"=0.0}, "ROOTMOOP1"={"Index"=29, "Value"=0.0}, "ROOTMOOP2"={"Index"=30, "Value"=0.0}, "BL_PITCH2"={"Index"=32, "Value"=0.0}, "BL_PITCH3"={"Index"=33, "Value"=0.0}, "ROOTMOOP3"={"Index"=31, "Value"=0.0}, "AVCMSG_SIZE"={"Index"=48, "Value"=0.0}, "INFILE_SIZE "={"Index"=49, "Value"=0.0}, "OUTFILE_SIZE "={"Index"=50, "Value"=0.0}, "FA_ACC"={"Index"=52, "Value"=0.0}, "NUM_BLADES"={"Index"=60, "Value"=0.0}, "OUT_BL_PITCH"={"Index"=44, "Value"=0.0}, "OUT_TORQUE"={"Index"=46, "Value"=0.0}, "OUT_AEROTQ"={"Index"=89, "Value"=0.0}, "Out.RotSpeed "={"Index"=92, "Value"=0.0}, "Out.DEBUG"={"Index"=93, "Value"=0.0}} ("ArrayPairs"), "GEN_SPEED.Value"=w329, "DT.Value"=sgl 0.001 ("Dt"), "AVCMSG_SIZE.Value"=sgl 65536.0 ("new element/subarray"), "INFILE_SIZE.Value"=sgl 33.0 ("new element/subarray"), "OUTFILE_SIZE.Value"=sgl 35.0 ("new element/subarray"), "BL_PITCH.Value"=w328, "ROTOR_SPEED.Value"=w327, "NUM_BLADES.Value"=sgl 3.0 ("NumberofBlades"), "GENTQMEAS.Value"=w325, "VS_GENPWR.Value"=w324) -> (w323:T5)
    n183 = shared-variable ".\\SharedVars.lvlib\\ArrayPairs"(w323) -> ()  [unwired: 1 in, 1 out]
    n184 = shared-variable ".\\SharedVars.lvlib\\StopLV"() -> (w335:bool)  [unwired: 1 in, 1 out]
    n185 = node-c288() -> ()  [unwired: 1 in, 1 out]
  }
  n186 = node-c288(w35) -> ()  [unwired: 1 out]
  n187 = node-c288(w39) -> ()  [unwired: 1 out]
  n188 = node-c288(w33) -> ()  [unwired: 1 out]
  n189 = node-c288(w43) -> ()  [unwired: 1 out]
  n190 = node-c288(w41) -> ()  [unwired: 1 out]
  n191 = node-c288(w37) -> ()  [unwired: 1 out]
  n192 = call <vilib>:"Simple Error Handler.vi"("error in (no error)"=w15) -> ()  [unwired: 4 in, 5 out]
  n193 = call <vilib>:"Simple Error Handler.vi"("error in (no error)"=w17) -> ()  [unwired: 4 in, 5 out]
